vi "GetSoundVeloc.vi"(8 "错误输入（无错误）":errorcluster) -> (0 "错误输出":errorcluster, 3 "返回值":u32)   [LabVIEW 2014]
uses:
  X86Dll/ZXUTConfigMgr.dll
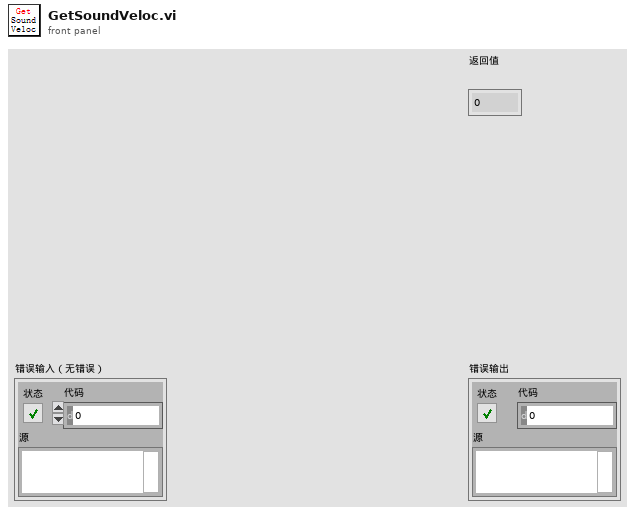
[diagram p1: front panel]
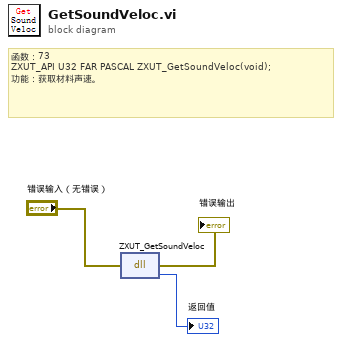
[diagram p0: block diagram]
diagram:
  # "函数：73\nZXUT_API U32\tFAR PASCAL ZXUT_GetSoundVeloc(void);\n功能：获取材料声速。"
  n1 = dll-call lib="D:/Software/Utrasonic on-line monitoring/X86Dll/ZXUTConfigMgr.dll" fn="ZXUT_GetSoundVeloc"(error in="错误输入（无错误）") -> (error out=→"错误输出":errorcluster, "返回值"=→"返回值":u32)  [unwired: 2 in, 1 out]
